vi "Panel.vi"(11 "Value Editor In":refnum<class "Value Editor Template.lvclass">) -> ()   [LabVIEW 2020, in "Value Editor Template.lvclass"]
uses:
  Value Editor Template.lvclass
  Value Editor Template.lvclass/Value Editor Template.ctl
  <vilib>/IlluminatedG/IG OOPanel/OOPanel/Panel/Basic UI State.ctl
  <vilib>/IlluminatedG/IG OOPanel/OOPanel/Panel/Panel.lvclass
  <vilib>/IlluminatedG/IG OOPanel/OOPanel/OOPanel.lvlib
  Value Editor Base/Value Editor Base.lvclass
  Element.ctl
  C:/dev/IlluminatedG/lv-FlexBlocks/Block/FlexBlocks/Value Editor Base/Value Editor Base.lvclass
  C:/Program Files (x86)/National Instruments/LabVIEW 2020/vi.lib/IlluminatedG/IG OOPanel/OOPanel/ArrayPanel/ArrayPanel.lvclass
  C:/Program Files (x86)/National Instruments/LabVIEW 2020/vi.lib/IlluminatedG/IG OOPanel/OOPanel/Panel/Panel.lvclass
  C:/dev/IlluminatedG/lv-FlexBlocks/Block/FlexBlocks/Value Editor Template/Value Editor Template.lvclass
  Terminal Mode.ctl
  FlexBlocks.lvlib
panel:
  in  "Element":T1 format="%.3p"
  in  "Terminal Type":T2
  out "Value Name":string
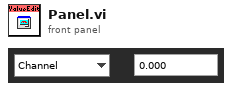
[diagram p1: front panel]
types:
  T1 = typedef "Value Editor Template.lvclass/Element.ctl" = dbl
  T2 = typedef "FlexBlocks.lvlib/Terminal Mode.ctl" = enum16{"Channel", "Config", "Value", "Control Ref"}
  T3 = typedef "OOPanel.lvlib/Panel.lvclass/Basic UI State.ctl" = enum16{"Init", "Run", "Close"}
  T4 = typedef "Value Editor Base.lvclass/Inbound Events.ctl" = cluster{"Update Type":refnum<user-event>, "Update Terminal":refnum<user-event>, "Update Value":refnum<user-event>}
  T5 = typedef "OOPanel.lvlib/Panel.lvclass/Panel Events.ctl" = cluster{"Visbility":refnum<user-event>, "Close":refnum<user-event>}
  T6 = typedef "FlexBlocks.lvlib/Type Descriptor.ctl" = cluster{"Name":string, "Direction":T7, "Default":variant, "Min":variant, "Max":variant, "Step":variant, "Value Mode":T8, "Required":bool, "Connpane Index":i32, "Special Terminal":T9, "Color":u32, "Options":string[], "Type String":string, "Sort":i32, "Item Path":path}
  T7 = typedef "FlexBlocks.lvlib/Terminal Direction.ctl" = enum16{"Sink", "Source"}
  T8 = typedef "FlexBlocks.lvlib/Value Mode.ctl" = enum16{"Normal", "Range", "Select"}
  T9 = typedef "FlexBlocks.lvlib/Special Terminal.ctl" = enum16{"None", "Action", "Init", "Tag", "State in", "State out", "Error"}
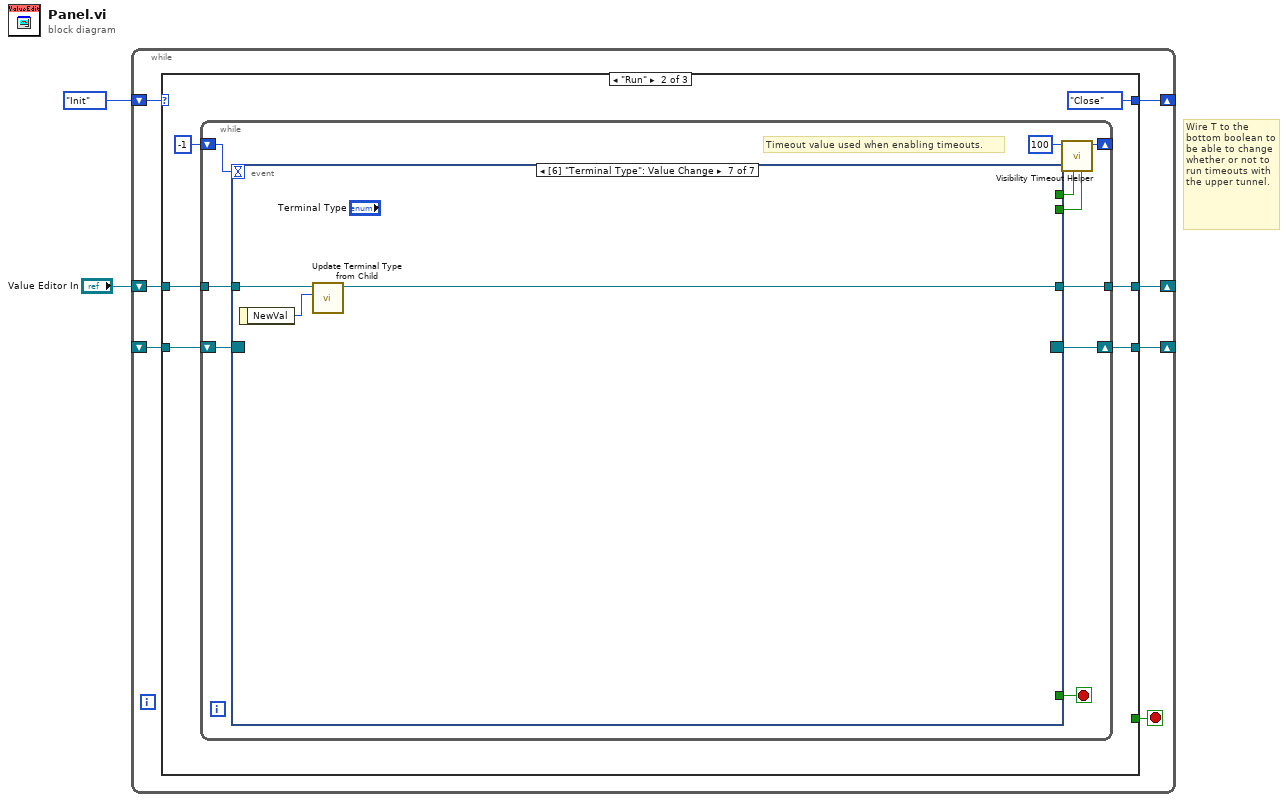
[diagram p0: block diagram]
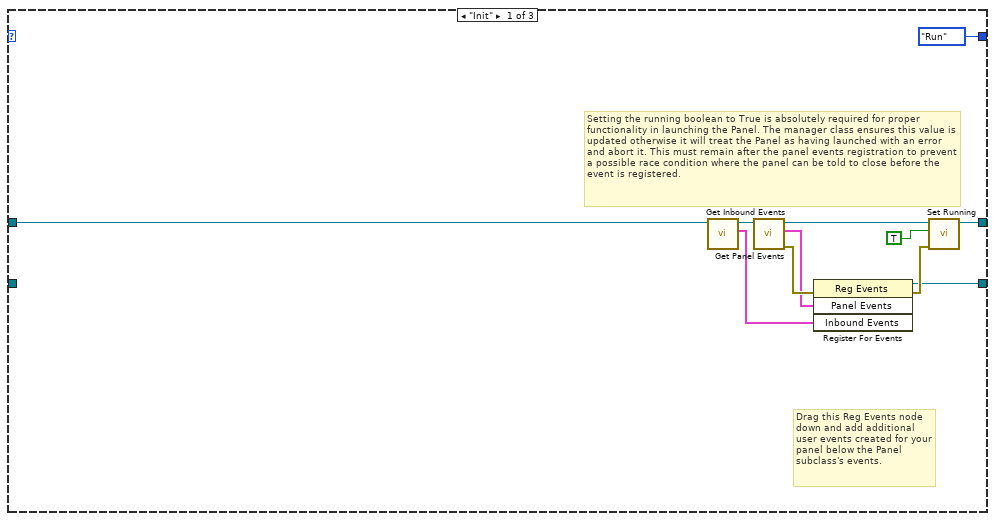
[diagram p2: hidden frame]
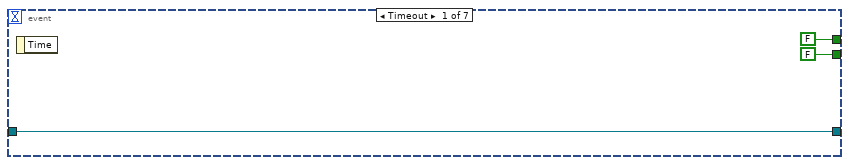
[diagram p3: hidden frame]
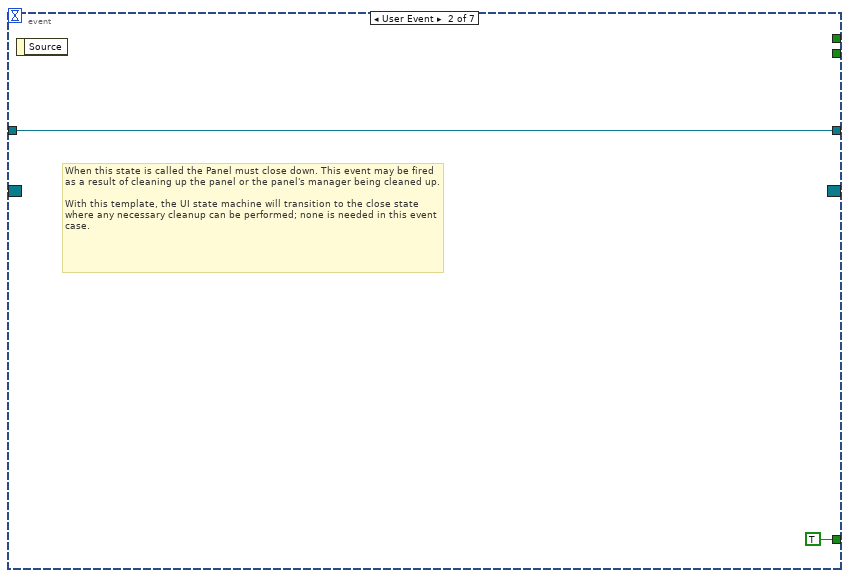
[diagram p4: hidden frame]
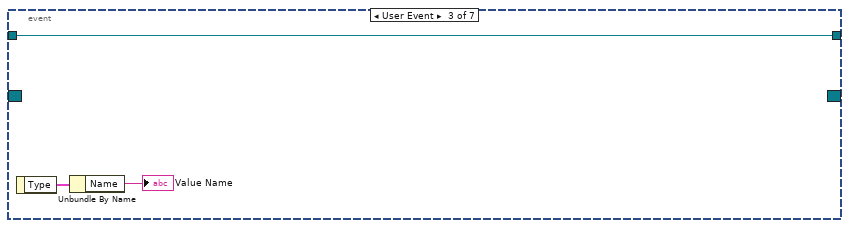
[diagram p5: hidden frame]
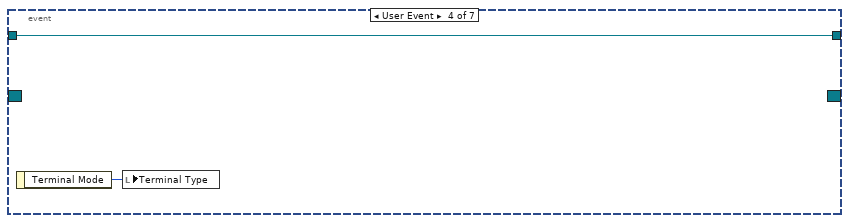
[diagram p6: hidden frame]
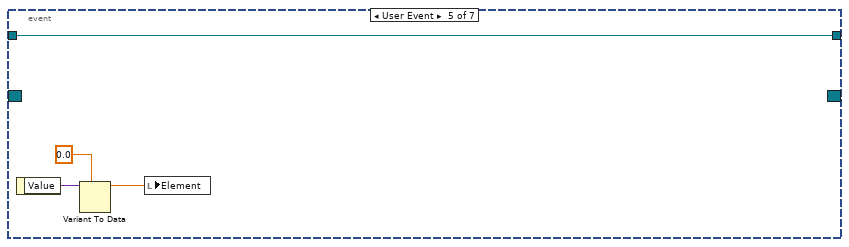
[diagram p7: hidden frame]
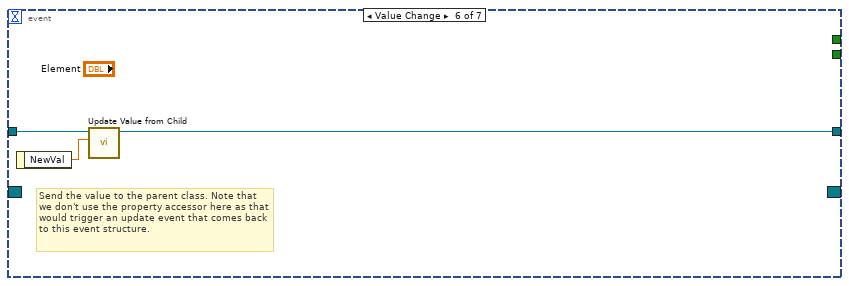
[diagram p8: hidden frame]
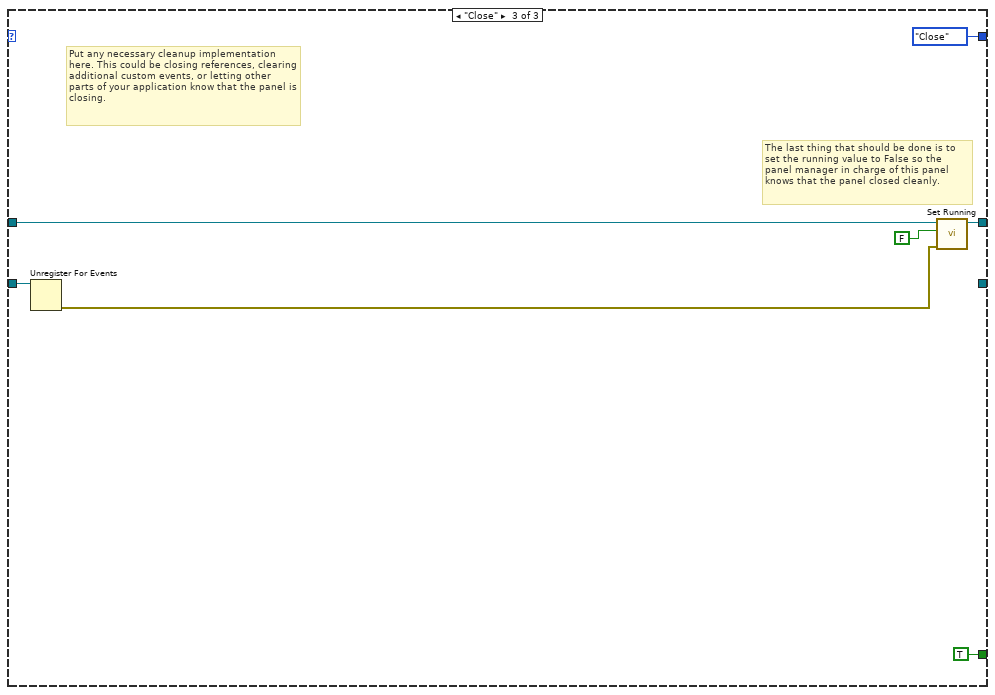
[diagram p9: hidden frame]
diagram:
  # "Wire T to the bottom boolean to be able to change whether or not to run timeouts with the upper tunnel."
  n1 = while {
    shift-right: [w8] -> _
    shift-left: _ -> [w9]
    shift-right: [w6] -> _
    shift-left: Basic_UI_State."Init" ("Basic UI State") -> [w7]
    shift-right: [w4] -> _
    shift-left: "Value Editor In" -> [w3]
    stop <- w5 stop-if-true
    n2 = case shown="\"Run\"" w7 {
      tunnel: w9 -> [_ w26 w59]
      tunnel: [w14 w24 _] -> w8
      tunnel: [Basic_UI_State."Run" ("Basic UI State") Basic_UI_State."Close" ("Basic UI State") Basic_UI_State."Close" ("Basic UI State")] -> w6
      tunnel: [_ _ TRUE] -> w5
      tunnel: [w13 w21 w57] -> w4
      tunnel: w3 -> [w11 w22 w58]
      frame "Init" {
        # "Setting the running boolean to True is absolutely required for proper functionality in launching the Panel. The manager class ensures this value is updated otherwise it will treat the Panel as having launched with an error and abort it. This must remain after the panel events registration to prevent a possible race condition where the panel can be told to close before the event is registered."
        # "Drag this Reg Events node down and add additional user events created for your panel below the Panel subclass's events."
        n3 = call "Get Inbound Events.vi"("Value Editor Base in"=w11) -> ("Inbound Events"=w10:T4, "Value Editor Base out"=w12:refnum<class "Value Editor Template.lvclass">)  [unwired: 8 in, 1 out]
        n4 = call <vilib>:"Get Panel Events.vi"("Panel in"=w12) -> ("error out"=w20:errorcluster, "Panel Events"=w16:T5, "Panel out"=w17:refnum<class "Value Editor Template.lvclass">)  [unwired: 8 in]
        n5 = register-events(error in=w20, w16, w10) -> (reference out=w14:refnum<event-registration>, error out=w18:errorcluster)  [unwired: 1 in]
        n6 = call <vilib>:"Set Running.vi"("error in (no error)"=w18, "Running"=TRUE, "Panel in"=w17) -> ("Panel out"=w13:refnum<class "Value Editor Template.lvclass">)  [unwired: 7 in, 1 out]
      }
      frame "Run" {
        n7 = while {
          shift-right: [w32] -> w24
          shift-left: w26 -> [w33]
          shift-right: [w35] -> _
          shift-left: -1 ("Timeout") -> [w34]
          tunnel: w22 -> [w28]
          tunnel: [w27] -> w21
          stop <- w29 stop-if-true
          # "Timeout value used when enabling timeouts."
          n8 = event shown="[6] \"Terminal Type\": Value Change" {
            selector: w33 -> [_ _ _ _ _ _ _]
            dyn-events: [_ _ _ _ _ _ _] -> w32
            timeout: w34 -> [_ _ _ _ _ _ _]
            tunnel: [FALSE _ _ _ _ _ _] -> w31
            tunnel: [FALSE _ _ _ _ _ _] -> w30
            tunnel: [_ TRUE _ _ _ _ _] -> w29
            tunnel: w28 -> [w37 w40 w42 w45 w47 w53 w56]
            tunnel: [w37 w40 w42 w45 w47 w51 w54] -> w27
            event Timeout {
              n9 = event-data() -> ()  [unwired: 1 in, 1 out]
            }
            event User Event {
              # "When this state is called the Panel must close down. This event may be fired as a result of cleaning up the panel or the panel's manager being cleaned up.\n\nWith this template, the UI state machine will transition to the close state where any necessary cleanup can be performed; none is needed in this event case."
              n10 = event-data() -> ()  [unwired: 1 in, 1 out]
            }
            event User Event {
              n11 = event-data() -> ("Type"=w44:T6)  [unwired: 1 in]
              n12 = Unbundle By Name(w44) -> ("Name"=→"Value Name":string)
            }
            event User Event {
              n13 = event-data() -> ("Terminal Mode"=w46:T2)  [unwired: 1 in]
              n14 = local write "Terminal Type"(w46) -> ()
            }
            event User Event {
              n15 = event-data() -> ("Value"=w50:variant)  [unwired: 1 in]
              n16 = Variant To Data(type=T1 0.0 ("Element"), Variant=w50) -> (data=w48:T1)  [unwired: 1 in, 1 out]
              n17 = local write "Element"(w48) -> ()
            }
            event Value Change {
              # "Send the value to the parent class. Note that we don't use the property accessor here as that would trigger an update event that comes back to this event structure."
              n18 = event-data() -> ("NewVal"=w52:T1)  [unwired: 1 in]
              n19 = call "Update Value from Child.vi"("Value"=w52, "Value Editor Base in"=w53) -> ("Value Editor Base out"=w51:refnum<class "Value Editor Template.lvclass">)  [unwired: 8 in, 1 out]
            }
            event Value Change {
              n20 = event-data() -> ("NewVal"=w55:T2)  [unwired: 1 in]
              n21 = call "Update Terminal Type from Child.vi"("Terminal Type"=w55, "Value Editor Base in"=w56) -> ("Value Editor Base out"=w54:refnum<class "Value Editor Template.lvclass">)  [unwired: 8 in, 1 out]
            }
          }
          n22 = call <vilib>:"Visibility Timeout Helper.vi"("Update?"=w30, "Use Timeout?"=w31, "Visible Timeout mS"=100) -> ("Timeout"=w35:i32)  [unwired: 8 in]
        }
      }
      frame "Close" {
        # "Put any necessary cleanup implementation here. This could be closing references, clearing additional custom events, or letting other parts of your application know that the panel is closing."
        # "The last thing that should be done is to set the running value to False so the panel manager in charge of this panel knows that the panel closed cleanly."
        n23 = Unregister For Events(event registration refnum=w59) -> (error out=w61:errorcluster)  [unwired: 1 in]
        n24 = call <vilib>:"Set Running.vi"("error in (no error)"=w61, "Running"=FALSE, "Panel in"=w58) -> ("Panel out"=w57:refnum<class "Value Editor Template.lvclass">)  [unwired: 7 in, 1 out]
      }
    }
  }
